vi "Update Status.vi"(8 "error in (no error)":errorcluster, 10 "Status":string, 11 "Worker in":refnum<class "Worker.lvclass">) -> (0 "error out":errorcluster, 3 "Worker out":refnum<class "Worker.lvclass">)   [LabVIEW 2020, in "Worker.lvclass"]
uses:
  Worker.lvclass
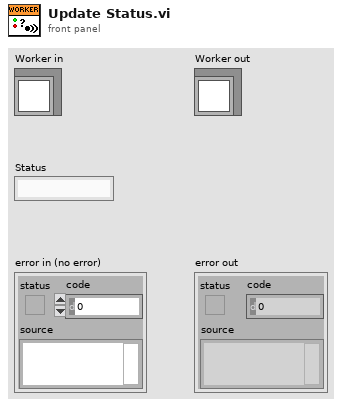
[diagram p1: front panel]
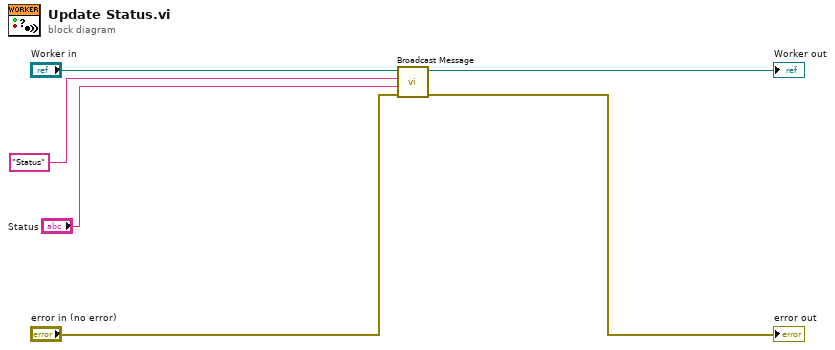
[diagram p0: block diagram]
diagram:
  n1 = call-dynamic "Broadcast Message.vi"("error in (no error)"="error in (no error)", "Message Data"="Status", "Message"="Status", "Rig Process In"="Worker in") -> ("error out"=→"error out":errorcluster, "Rig Process Out"=→"Worker out":refnum<class "Worker.lvclass">)  [unwired: 6 in]
